vi "Read Calibration Breakpoints 340 Format.vi"(0 "Calibration File":path=path "C:/User/Brand/LVP/CSPP-Dev/Packages/LS218/X42700.txt", 11 "Error In":errorcluster) -> (2 "Temp Coefficient":u16(ring) items=["Negative", "Positive"], 3 "Curve Data Format":u16(ring) items=["V/K", "Ohms/K", "Log Ohms/K"], 6 "Curve Name":string, 8 "Curve Serial Number":string, 10 "Limit Value":dbl=475.0 min=0.0 max=999.99 step=0.01 format="%.2f", 14 "Calibration Points":T1(array[cluster]), 15 "Error Out":errorcluster)   [LabVIEW 2013, in "LS218.lvlib" / "LS218.lvclass"]
doc: "Read calibration curve from file with BREAKPOINTS 340 FORMAT."
uses:
  LS218.lvclass
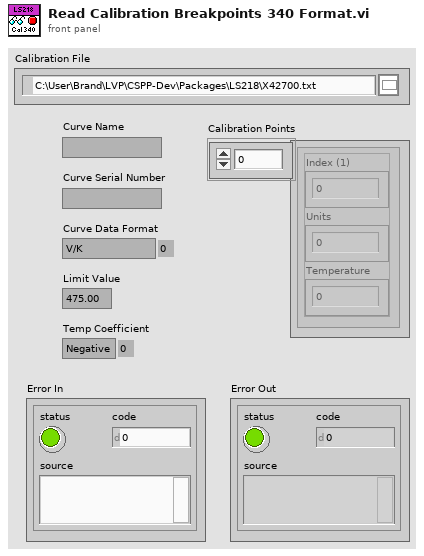
[diagram p1: front panel]
types:
  T1 = cluster{"Index (1)":i32, "Units":dbl, "Temperature":dbl}[]
  T2 = enum16{"open", "replace", "create", "open or create", "replace or create", "replace or create with confirmation"}
  T3 = cluster{"Index (1)":i32, "Units":dbl, "Temperature":dbl}
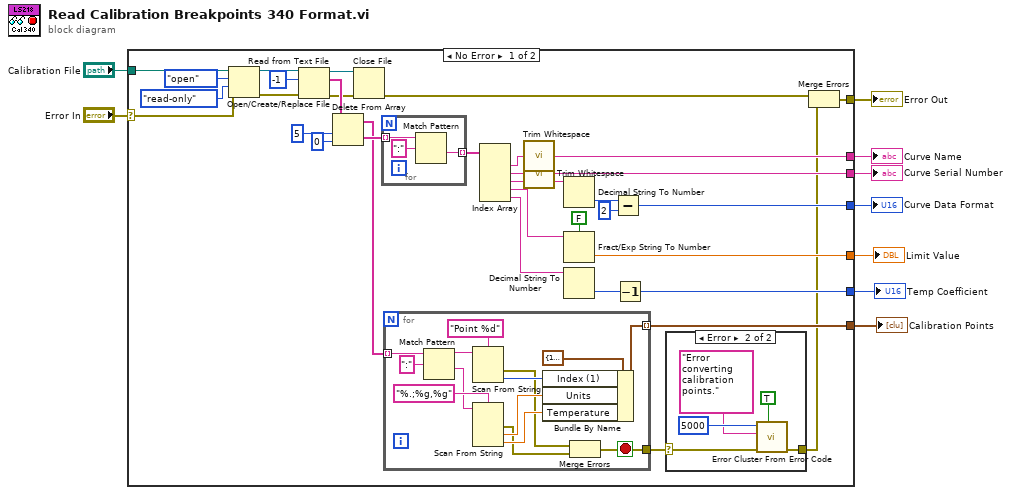
[diagram p0: block diagram]
diagram:
  n1 = case shown="No Error" "Error In" {
    selector: "Error In" -> [w13 w67]
    tunnel: "Calibration File" -> [w21 _]
    tunnel: [w20 _] -> w8
    tunnel: [w19 _] -> w7
    tunnel: [w18 _] -> w6
    tunnel: [w17 _] -> w5
    tunnel: [w16 _] -> w4
    tunnel: [w11 w67] -> w3
    tunnel: [w14 _] -> w2
    frame No Error {
      n2 = Open/Create/Replace File(file path (use dialog)=w21, error in=w13, operation (0:open)=T2."open", access (0:read/write)=enum16{"read/write", "read-only", "write-only"}."read-only") -> (refnum out=w40:refnum<file>, error out=w41:errorcluster)  [unwired: 2 in, 1 out]
      n3 = Read from Text File(file (use dialog)=w40, count=-1, error in=w41) -> (refnum out=w37:refnum<file>, text=w38:string[], error out=w36:errorcluster)  [unwired: 1 in, 1 out]
      n4 = Delete From Array(array=w38, length=5, index=0) -> (deleted portion=w34:string[], array with subset deleted=w22:string[])
      n5 = Close File(refnum=w37, error in=w36) -> (error out=w15:errorcluster)  [unwired: 1 out]
      n6 = for {
        tunnel: w34 -> [w66] mode=indexing
        tunnel: [w64] -> w33 mode=indexing
        n7 = Match Pattern(string=w66, regular expression=":") -> (after substring=w64:string)  [unwired: 1 in, 3 out]
      }
      n8 = for {
        tunnel: w22 -> [w54] mode=indexing
        tunnel: [w53] -> w14 mode=indexing
        tunnel: [w50] -> w12
        stop <- w50 stop-if-true
        n9 = Match Pattern(string=w54, regular expression=":") -> (before substring=w62:string, after substring=w60:string)  [unwired: 1 in, 2 out]
        n10 = Scan From String(format string="Point %d", input string=w62) -> (error out=w52:errorcluster, output 1=w57:i32)  [unwired: 3 in, 2 out]
        n11 = Scan From String(format string="%.;%g,%g", input string=w60) -> (error out=w51:errorcluster, output 1=w56:dbl, output 2=w55:dbl)  [unwired: 4 in, 2 out]
        n12 = Bundle By Name(cluster=T3 {"Index (1)"=1, "Units"=0.0, "Temperature"=0.0} ("Calibration Point"), "Index (1)"=w57, "Units"=w56, "Temperature"=w55) -> (w53:T3)
        n13 = Merge Errors(w52, w51) -> (w50:errorcluster)
      }
      n14 = Index Array(array=w33) -> (element #1=w32:string, element #2=w31:string, element #3=w30:string, element #4=w25:string, element #5=w26:string)  [unwired: 5 in]
      n15 = call <vilib>:"Trim Whitespace.vi"("string"=w32) -> ("trimmed string"=w20:string)  [unwired: 1 in]
      n16 = call <vilib>:"Trim Whitespace.vi"("string"=w31) -> ("trimmed string"=w19:string)  [unwired: 1 in]
      n17 = Decimal String To Number(string=w30) -> (number=w29:i32)  [unwired: 2 in, 1 out]
      n18 = Fract/Exp String To Number(use system decimal point (T)=FALSE, string=w25) -> (number=w17:dbl)  [unwired: 2 in, 1 out]
      n19 = Decimal String To Number(string=w26) -> (number=w27:i32)  [unwired: 2 in, 1 out]
      n20 = Subtract(x=w29, y=2) -> (x-y=w18:i32)
      n21 = Decrement(x=w27) -> (x-1=w16:i32)
      n22 = case shown="Error" w12 {
        selector: w12 -> [w44 w49]
        tunnel: [w44 w48] -> w10
        frame No Error {
        }
        frame Error {
          n23 = call <vilib>:"Error Cluster From Error Code.vi"("show call chain? (False)"=TRUE, "error in (no error)"=w49, "error message (\"\")"="Error converting calibration points." ("error message (\"\")"), "error code (0)"=5000) -> ("error out"=w48:errorcluster)  [unwired: 5 in]
        }
      }
      n24 = Merge Errors(w15, w10) -> (w11:errorcluster)
    }
    frame Error {
    }
  }
  "Temp Coefficient" <- w4
  "Curve Data Format" <- w6
  "Limit Value" <- w5
  "Curve Name" <- w8
  "Curve Serial Number" <- w7
  "Error Out" <- w3
  "Calibration Points" <- w2
